vi "NTPModify.vi"() -> ()   [LabVIEW 2023]
uses:
  <vilib>/Utility/file.llb/Write Delimited Spreadsheet (I64).vi
panel:
  in  "Matches Tab":enum32{"Page 1", "Page 2"}(tab)
  out "Table Control":string[][](table)
  out "Data file (checkRes.txt, matches.txt, toto.txt):":path=path "/Users/blagojnikolov/Desktop/@tmp/checkRes.txt"
  in  "Time Ctr":bool
  out "appended array":string[](array[string])
  out "Average by row":u64[](array[numeric]) format="%-2.0f"
  out "Deviation by row":i64[][](array[numeric])
  in  "Last Draw":i64[](array[numeric])
  out "Matches":i32[][](array[numeric])
  out "Matches":i32[](array[numeric])
  out "Last Suppose":i32[][](array[numeric])
  out "?":bool
  in  "Deviation":bool
  in  "Check":bool
  in  "Play":bool
  out "Your Suppose":i32[][](array[numeric])
  out "Waveform Chart":i64[][](graph)
  in  "Stop":bool
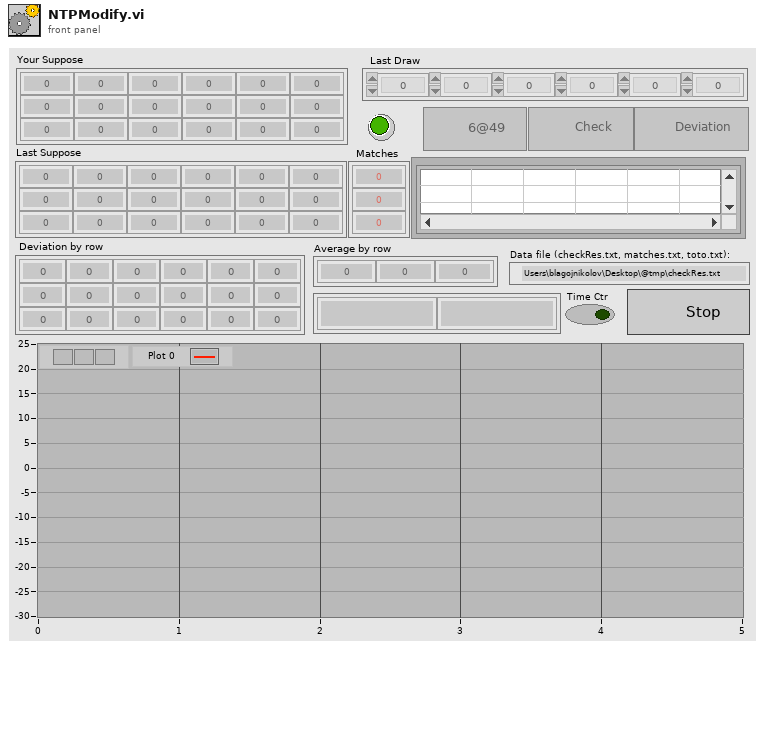
[diagram p1: front panel]
types:
  T1 = enum8{"Enabled", "Disabled", "Disabled and Grayed Out"}
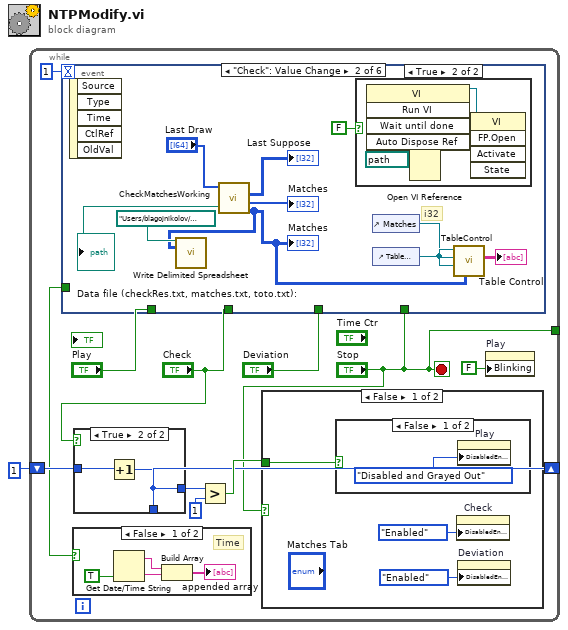
[diagram p0: block diagram]
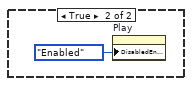
[diagram p4: hidden frame]
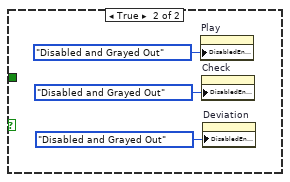
[diagram p5: hidden frame]
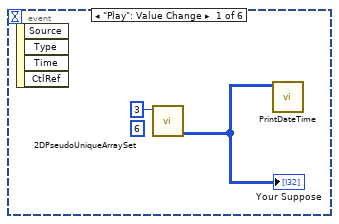
[diagram p6: hidden frame]
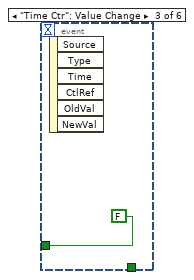
[diagram p8: hidden frame]
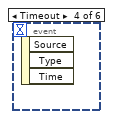
[diagram p9: hidden frame]
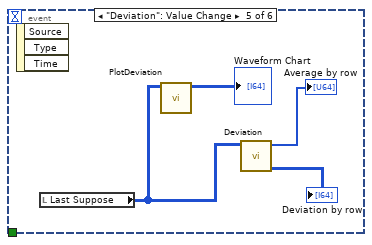
[diagram p10: hidden frame]
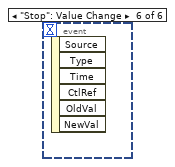
[diagram p11: hidden frame]
diagram:
  n1 = while {
    shift-right: [w6] -> _
    shift-left: i64 1 -> [w8]
    tunnel: ["Stop"] -> _
    stop <- "Stop" stop-if-true
    n2 = event shown="[1] \"Check\": Value Change" {
      selector: _ -> [_ _ _ _ _ _]
      dyn-events: _ -> [_ _ _ _ _ _]
      timeout: 1 -> [_ _ _ _ _ _]
      tunnel: "Play" -> [_ _ _ _ _ _]
      tunnel: "Check" -> [_ _ _ _ _ _]
      tunnel: "Deviation" -> [_ _ _ _ _ _]
      tunnel: "Stop" -> [_ _ _ _ _ _]
      tunnel: [_ _ FALSE _ _ _] -> w2
      event "Play": Value Change {
        (unwired) 6 ("Colums")
        n3 = event-data() -> ()  [unwired: 1 in, 4 out]
        n4 = call "2DPseudoUniqueArraySet.vi"("Rows"=3) -> ("2D Double Array"=w29:i32[][])  [unwired: 9 in, 1 out]
        "Your Suppose" <- w29
        n5 = call "PrintDateTime.vi"("2D Double"=w29) -> ()  [unwired: 10 in, 1 out]
      }
      event "Check": Value Change {
        # "i32"
        n6 = event-data() -> ()  [unwired: 1 in, 5 out]
        n7 = call "CheckMatchesWorking.vi"("Последен тираж"="Last Draw") -> (0:w35:i64[][], "Съвпадения"=→"Matches":i32[], "Залози"=→"Last Suppose":i32[][], "file path (dialog if empty)"=→"Data file (checkRes.txt, matches.txt, toto.txt):":path)  [unwired: 7 in]
        "Matches" <- w35
        n8 = call-poly <vilib>:"Write Delimited Spreadsheet.vi"("file path (dialog if empty)"=path "/Users/blagojnikolov/Desktop/@tmp/matches.txt", "2D data"=w35) -> ()  [unwired: 12 in, 2 out]
        n9 = case shown="True" FALSE {
          frame False {
          }
          frame True {
            n10 = Open VI Reference(vi path=path "/Users/blagojnikolov/Library/Mobile Documents/com~apple~CloudDocs/» LabView/LabView/Project'24/Projects/649/subVI Tools/CollorCellsInTableOnly.vi") -> (vi reference=w42:refnum<vi>)  [unwired: 5 in, 1 out]
            n11 = invoke on="Invoke Node" class="VI" method="Run VI"(reference=w42) -> (reference out=w41:refnum<vi>)  [unwired: 4 in, 4 out]
            n12 = invoke on="Invoke Node" class="VI" method="FP.Open"(reference=w41) -> ()  [unwired: 4 in, 5 out]
          }
        }
        n13 = control-ref of="Matches"() -> (w32:refnum<vi>)
        n14 = control-ref of="Table Control"() -> (w34:refnum<vi>)
        n15 = call "TableControl.vi"("2D Double Array"=w35, "Table Control in"=w34, "Arr Refnum"=w32, "Table in"=w34) -> ("Array"=→"Table Control":string[][])  [unwired: 7 in]
      }
      event "Time Ctr": Value Change {
        n16 = event-data() -> ()  [unwired: 1 in, 6 out]
      }
      event Timeout {
        n17 = event-data() -> ()  [unwired: 1 in, 3 out]
      }
      event "Deviation": Value Change {
        n18 = event-data() -> ()  [unwired: 1 in, 3 out]
        n19 = local read "Last Suppose"() -> (w46:i32[][])
        n20 = call "PlotDeviation.vi"("Array"=w46) -> ("Waveform Chart"=→"Waveform Chart":i64[][])  [unwired: 8 in, 2 out]
        n21 = call "Deviation.vi"("2D  Array"=w46) -> ("Deviation by row"=→"Deviation by row":i64[][], "Average in row"=→"Average by row":u64[])  [unwired: 9 in]
      }
      event "Stop": Value Change {
        n22 = event-data() -> ()  [unwired: 1 in, 6 out]
      }
    }
    n23 = case shown="False" w2 {
      frame False {
        # "Time"
        n24 = Get Date/Time String(want seconds? (F)=TRUE) -> (date string=w15:string, time string=w16:string)  [unwired: 2 in]
        n25 = Build Array(w15, w16) -> (→"appended array":string[])
      }
      frame True {
      }
    }
    n26 = case shown="True" "Check" {
      tunnel: [w18 w19] -> w7
      tunnel: [w18 w19] -> w6
      tunnel: w8 -> [w18 w20]
      frame False {
      }
      frame True {
        n27 = Increment(x=w20) -> (x+1=w19:i64)
      }
    }
    n28 = Greater?(x=w7, y=i64 1) -> (0:w9:bool)
    n29 = case shown="False" "Stop" {
      tunnel: w9 -> [w21 _]
      frame False {
        n30 = case shown="False" w21 {
          frame False {
            n31 = property on="Play" class="Bool"("DisabledEnum"=T1."Disabled and Grayed Out" ("Disabled")) -> ()  [unwired: 2 in, 2 out]
          }
          frame True {
            n32 = property on="Play" class="Bool"("DisabledEnum"=T1."Enabled" ("Disabled")) -> ()  [unwired: 2 in, 2 out]
          }
        }
        n33 = property on="Check" class="Bool"("DisabledEnum"=T1."Enabled" ("Disabled")) -> ()  [unwired: 2 in, 2 out]
        n34 = property on="Deviation" class="Bool"("DisabledEnum"=T1."Enabled" ("Disabled")) -> ()  [unwired: 2 in, 2 out]
      }
      frame True {
        n35 = property on="Play" class="Bool"("DisabledEnum"=T1."Disabled and Grayed Out" ("Disabled")) -> ()  [unwired: 2 in, 2 out]
        n36 = property on="Check" class="Bool"("DisabledEnum"=T1."Disabled and Grayed Out" ("Disabled")) -> ()  [unwired: 2 in, 2 out]
        n37 = property on="Deviation" class="Bool"("DisabledEnum"=T1."Disabled and Grayed Out" ("Disabled")) -> ()  [unwired: 2 in, 2 out]
      }
    }
    n38 = property on="Play" class="Bool"("Blinking"=FALSE) -> ()  [unwired: 2 in, 2 out]
  }
